vi "Variant From Registry.vi"(4 "Registry Variant Accessor in":refnum<class "CConfig Variant Accessor.lvclass">, 5 "Strip Whitespace? [T]":bool=TRUE, 7 "Variant":variant, 8 "error in (no error)":errorcluster, 9 "Use LV Default? [F]":bool, 11 "Carya Config in":refnum<class "Carya Config.lvclass">) -> (0 "error out":errorcluster, 1 "Set?":bool, 2 "Variant":variant, 3 "Carya Config out":refnum<class "Carya Config.lvclass">)   [LabVIEW 2013, in "Carya Config.lvclass"]
doc: "Copyright 2018, Carya Automatisering, Wiebe Walstra."
uses:
  Carya Config.lvclass
  CConfig Variant Accessor/CConfig Variant Accessor.lvclass
  CConfig Variant Accessor/CConfig Variant Accessor.lvclass/CConfig Variant Accessor.ctl
  <vilib>/Utility/error.llb/Error Cluster From Error Code.vi
  <vilib>/ErrorRing/Error Ring.xnode
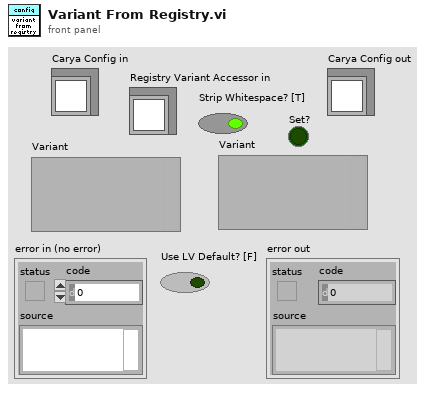
[diagram p1: front panel]
types:
  T1 = typedef "VariantType.lvlib/Type.ctl" = enum8{"Invalid Type", "Void", "I8", "I16", "I32", "I64", "U8", "U16", "U32", "U64", "Single Float", "Double Float", "Extended Float", "Single Complex", "Double Complex", "Extended Complex", "Enum U8", "Enum U16", "Enum U32", "Enum U64", "Single Float With Unit", "Double Float With Unit", "Extended Float With Unit", "Single Complex with Unit", "Double Complex with Unit", "Extended Complex with Unit", "Boolean", "String", "Path", "Picture", "Tag", "Array", "Cluster", "Variant", "LV Variant", "Waveform", "Timestamp", "Digital Waveform", "Digital Data", "ExpressData", "Refnum", "External Data", "VI", "Poly VI", "LabVIEW Class Instance", "Fixed Point"}
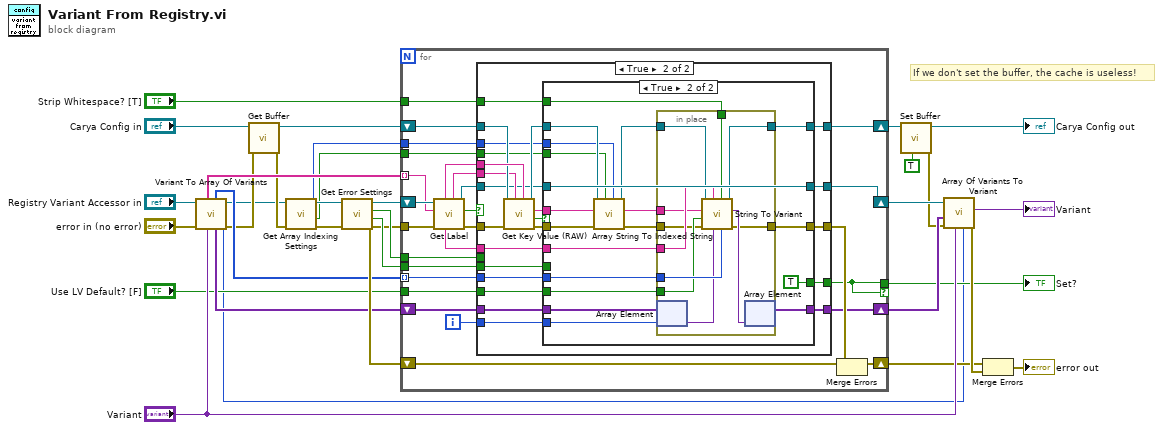
[diagram p0: block diagram]
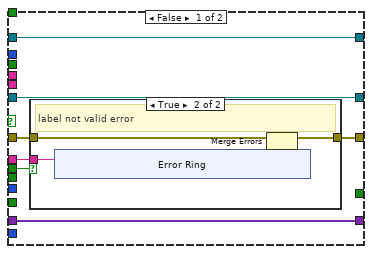
[diagram p2: hidden frame]
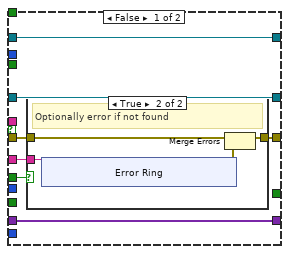
[diagram p4: hidden frame]
diagram:
  # "If we don't set the buffer, the cache is useless!"
  n1 = call-dynamic "Variant To Array Of Variants.vi"("Variant"="Variant", "error in (no error)"="error in (no error)", "Registry Variant Accessor in"="Registry Variant Accessor in") -> ("error out"=w12:errorcluster, "Type Enum [auto]"=w7:T1, "Registry Variant Accessor out"=w4:refnum<class "CConfig Variant Accessor.lvclass">, "Variants"=w24:variant[], "Types"=w25:T1[], "Labels (RAW)"=w23:string[])  [unwired: 3 in]
  n2 = call-dynamic "Get Buffer.vi"("error in (no error)"=w12, "Carya Config in"="Carya Config in") -> ("error out"=w15:errorcluster, "Config"=w11:refnum<class "Carya Config.lvclass">)  [unwired: 8 in]
  n3 = call "Get Array Indexing Settings.vi"("error in (no error)"=w15, "CConfig Variant Accessor in"=w4) -> ("error out"=w5:errorcluster, "Array indexing"=w1:bool, "Index"=w2:i32, "CConfig Variant Accessor out"=w3:refnum<class "CConfig Variant Accessor.lvclass">)  [unwired: 6 in]
  n4 = call "Get Error Settings.vi"("error in (no error)"=w5, "CConfig Variant Accessor in"=w3) -> ("error out"=w26:errorcluster, "Key not found error"=w28:bool, "Wrong label error"=w29:bool, "CConfig Variant Accessor out"=w27:refnum<class "CConfig Variant Accessor.lvclass">)  [unwired: 6 in]
  n5 = for {
    tunnel: w29 -> [w59]
    tunnel: w28 -> [w58]
    tunnel: w26 -> [w56]
    shift-right: [w52] -> w10
    shift-left: w11 -> [w53]
    shift-right: [w49] -> w16
    shift-left: w26 -> [w51]
    tunnel: w25 -> [w48] mode=indexing
    tunnel: w23 -> [w46] mode=indexing
    shift-right: [w36] -> w22
    shift-left: w27 -> [w57]
    tunnel: "Use LV Default? [F]" -> [w44]
    tunnel: [w43] -> w9 if=w43
    tunnel: "Strip Whitespace? [T]" -> [w42]
    shift-right: [w45] -> w20
    shift-left: w24 -> [w47]
    tunnel: w2 -> [w35]
    tunnel: w1 -> [w34]
    i -> [w41]
    n6 = call-dynamic "Get Label.vi"("error in (no error)"=w56, "Label"=w46, "Registry Variant Accessor in"=w57) -> ("error out"=w54:errorcluster, "Valid?"=w38:bool, "Registry Variant Accessor out"=w37:refnum<class "CConfig Variant Accessor.lvclass">, "Section out"=w40:string, "Complete label"=w55:string, "Key out"=w39:string)  [unwired: 3 in]
    n7 = case shown="True" w38 {
      tunnel: [w63 w101] -> w50
      tunnel: [w66 w100] -> w52
      tunnel: w47 -> [w65 w99]
      tunnel: [w65 w98] -> w45
      tunnel: w54 -> [w64 w93]
      tunnel: w39 -> [_ w92]
      tunnel: w53 -> [w66 w91]
      tunnel: w55 -> [w62 w90]
      tunnel: w48 -> [_ w89]
      tunnel: w59 -> [w61 _]
      tunnel: w58 -> [_ w88]
      tunnel: w44 -> [_ w87]
      tunnel: [_ w86] -> w43
      tunnel: w42 -> [_ w85]
      tunnel: w41 -> [_ w84]
      tunnel: w40 -> [_ w83]
      tunnel: w37 -> [w60 w82]
      tunnel: [w60 w81] -> w36
      tunnel: w35 -> [_ w80]
      tunnel: w34 -> [_ w79]
      frame False {
        n8 = case shown="True" w61 {
          tunnel: w64 -> [w67 w70]
          tunnel: [w67 w69] -> w63
          tunnel: w62 -> [_ w68]
          frame False {
            # "Ignore label not valid"
          }
          frame True {
            # "label not valid error"
            n9 = xnode "Error Ring"("parameter 0"=w68) -> ("error out"=w71:errorcluster)
            n10 = Merge Errors(w70, w71) -> (w69:errorcluster)
          }
        }
      }
      frame True {
        n11 = call-dynamic "Get Key Value (RAW).vi"("Key name"=w92, "Section name"=w83, "error in (no error)"=w93, "Carya Config in"=w91) -> ("error out"=w97:errorcluster, "Found?"=w94:bool, "Value"=w95:string, "Carya Config out"=w96:refnum<class "Carya Config.lvclass">)  [unwired: 4 in]
        n12 = case shown="True" w94 {
          tunnel: [w103 w128] -> w101
          tunnel: [w108 w139] -> w100
          tunnel: w90 -> [w105 w138]
          tunnel: w99 -> [w107 w133]
          tunnel: [w107 w132] -> w98
          tunnel: w97 -> [w106 w129]
          tunnel: w96 -> [w108 w126]
          tunnel: w95 -> [_ w124]
          tunnel: w89 -> [_ w137]
          tunnel: w88 -> [w104 _]
          tunnel: w87 -> [_ w136]
          tunnel: [_ TRUE] -> w86
          tunnel: w85 -> [_ w134]
          tunnel: w84 -> [_ w131]
          tunnel: [w102 w130] -> w81
          tunnel: w82 -> [w102 w130]
          tunnel: w80 -> [_ w122]
          tunnel: w79 -> [_ w121]
          frame False {
            n13 = case shown="True" w104 {
              tunnel: w106 -> [w109 w112]
              tunnel: [w109 w111] -> w103
              tunnel: w105 -> [_ w110]
              frame False {
                # "Ignore key not found"
              }
              frame True {
                # "Optionally error if not found"
                n14 = xnode "Error Ring"("parameter 0"=w110) -> ("error out"=w113:errorcluster)
                n15 = Merge Errors(w112, w113) -> (w111:errorcluster)
              }
            }
          }
          frame True {
            n16 = call-dynamic "Array String To Indexed String.vi"("Index [0]"=w122, "Array indexing [T]"=w121, "error in (no error)"=w129, "String (RAW)"=w124, "Registry Object"=w126) -> ("error out"=w127:errorcluster, "String"=w123:string, "Registry Object"=w125:refnum<class "Carya Config.lvclass">)  [unwired: 4 in]
            n17 = in-place {
              in-place-border: [w150] -> w139
              in-place-border: w138 -> [w149]
              in-place-border: w125 -> [w148]
              in-place-border: w123 -> [w147]
              in-place-border: w137 -> [w146]
              in-place-border: w136 -> [w142]
              in-place-border: w134 -> [w145]
              in-place-border: w127 -> [w141]
              in-place-border: [w140] -> w128
              n18 = in-place-array #1(w133, w131) -> (w144:variant)
              n19 = call-dynamic "String To Variant.vi"("Type Enum [auto]"=w146, "Strip Whitespace? [T]"=w145, "Variant Type\\default"=w144, "Name (error)"=w149, "error in (no error)"=w141, "Use LV Default? [F]"=w142, "String"=w147, "Registry Object"=w148) -> ("error out"=w140:errorcluster, "Variant"=w143:variant, "Registry Object"=w150:refnum<class "Carya Config.lvclass">)  [unwired: 1 in]
              n20 = in-place-array #1(w143) -> (w132:variant[])  [unwired: 1 out]
            }
          }
        }
      }
    }
    n21 = Merge Errors(w51, w50) -> (w49:errorcluster)
  }
  "Set?" <- w9
  n22 = call-dynamic "Set Buffer.vi"("Set? [T]"=TRUE, "Carya Config"=w10) -> ("error out"=w14:errorcluster, "Carya Config out"=→"Carya Config out":refnum<class "Carya Config.lvclass">)  [unwired: 8 in]
  n23 = call-dynamic "Array Of Variants To Variant.vi"("Type Enum [auto]"=w7, "Variant"="Variant", "error in (no error)"=w14, "Elements"=w20, "Registry Variant Accessor in"=w22) -> ("error out"=w18:errorcluster, "Variant"=→"Variant":variant)  [unwired: 4 in, 1 out]
  n24 = Merge Errors(w16, w18) -> (→"error out":errorcluster)
